vi "ST Motors.vi"(3 "error in (error out)":errorcluster, 4 "Motor State":string(combo)="OFF", 5 "VISA resource name in":refnum<visa-resource-name>) -> (0 "error out":errorcluster, 1 "SESSION \nENDED":bool, 2 "VISA resource name out":refnum<visa-resource-name>)   [LabVIEW 2009]
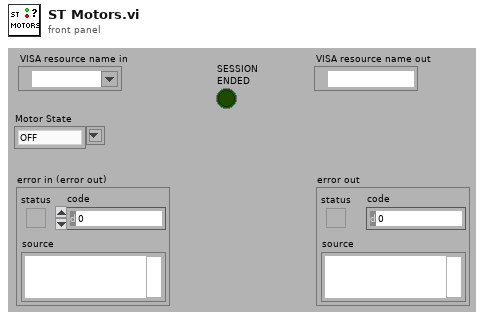
[diagram p1: front panel]
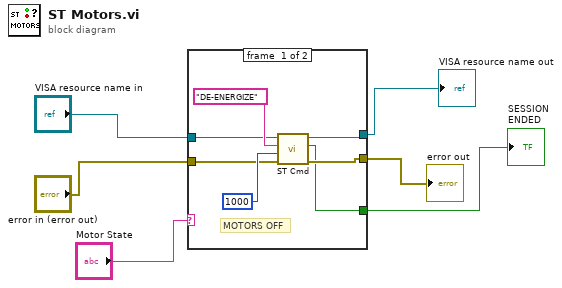
[diagram p0: block diagram]
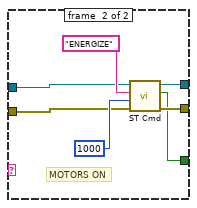
[diagram p2: hidden frame]
diagram:
  n1 = case shown="\"OFF\", Default" "Motor State" {
    tunnel: [w9 w20] -> w6
    tunnel: [w8 w19] -> w5
    tunnel: [w7 w18] -> w1
    tunnel: "VISA resource name in" -> [w11 w15]
    tunnel: "error in (error out)" -> [w10 w14]
    frame #0 {
      # "MOTORS OFF"
      n2 = call "ST Cmd.vi"("error in (no error)"=w10, "Time Out"=1000, "Command String"="DE-ENERGIZE", "VISA resource name"=w11) -> ("error out"=w8:errorcluster, "Ready and OK"=w7:bool, "VISA resource name out"=w9:refnum<visa-resource-name>)  [unwired: 2 out]
    }
    frame #1 {
      # "MOTORS ON"
      n3 = call "ST Cmd.vi"("error in (no error)"=w14, "Time Out"=1000, "Command String"="ENERGIZE", "VISA resource name"=w15) -> ("error out"=w19:errorcluster, "Ready and OK"=w18:bool, "VISA resource name out"=w20:refnum<visa-resource-name>)  [unwired: 2 out]
    }
  }
  "VISA resource name out" <- w6
  "error out" <- w5
  "SESSION \nENDED" <- w1
